vi "Name_Selector.vi"(11 "Path":string) -> (3 "Name":string)   [LabVIEW 2014]
panel:
  out "Array":string[](array[string])
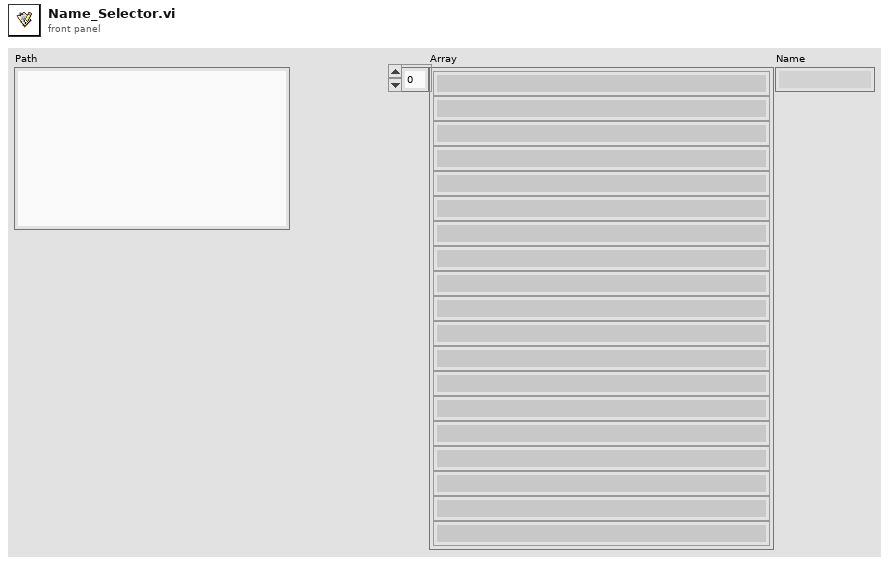
[diagram p1: front panel]
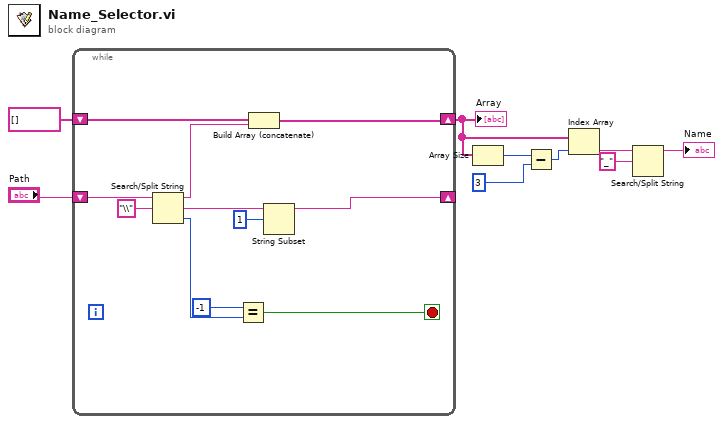
[diagram p0: block diagram]
diagram:
  n1 = while {
    shift-right: [w15] -> _
    shift-left: "Path" -> [w18]
    shift-right: [w12] -> w4
    shift-left: string[] [] -> [w11]
    stop <- w19 stop-if-true
    n2 = Search/Split String(string=w18, search string/char (-)="\\") -> (substring before match=w13:string, match + rest of string=w16:string, offset of match=w20:i32)  [unwired: 1 in]
    n3 = Equal?(x=-1, y=w20) -> (x = y?=w19:bool)
    n4 = Build Array (concatenate)(w11, w13) -> (w12:string[])
    n5 = String Subset(string=w16, offset (0)=1) -> (substring=w15:string)  [unwired: 1 in]
  }
  "Array" <- w4
  n6 = Array Size(array=w4) -> (size(s)=w7:i32)
  n7 = Subtract(x=w7, y=3) -> (x-y=w5:i32)
  n8 = Index Array(array=w4, index=w5) -> (element=w2:string)
  n9 = Search/Split String(string=w2, search string/char (-)="_") -> (substring before match=→"Name":string)  [unwired: 1 in, 2 out]
